vi "Modbus_RTU_Read.vi"(0 "VISA resource name":refnum<visa-resource-name>="COM18", 1 "Serial Config":T1={"baud rate (bps)"=9600, "stop bits"=10, "parity"=0, "flow control"=0, "timeout"=1000, "retries"=1} {"stop bits" items=["1.0"=10, "1.5"=15, "2.0"=20]; "parity" items=["None", "Odd", "Even", "Mark", "Space"]; "flow control" items=["None", "XON/XOFF", "RTS/CTS", "XON/XOFF & RTS/CTS", "DTR/DSR", "XON/XOFF & DTR/DSR"]}, 2 "address":u16=1, 4 "Registers In":u16[](array[numeric])=[1, 0, 2, 0, 0, 0, 0, 0, 0, 9], 5 "error in (no error)":errorcluster, 6 "Function":T2=enum."Read Holding Register03", 7 "Coil Single value":bool=TRUE, 8 "quantity":u16=2, 9 "Register Single Value":u16=100) -> (16 "VALUE":dbl, 19 "error out":errorcluster={"status"=FALSE, "code"=-1073807339, "source"="VISA Read in MB Master.lvlib:MB_ADU_RTU.lvclass:RX ADU.vi:4960001->MB Master.lvlib:MB_Master_Serial.lvclass:Querry.vi:3550001->MB Master.lvlib:Read Holding Registers.vi:2420001->Modbus_RTU_Setting.vi"})   [LabVIEW 2024]
uses:
  Modbus Control.ctl
  <vilib>/Plasmionique/MB Master/MB_Master_Serial/MB_Master_Serial.lvclass
  C:/Program Files (x86)/National Instruments/LabVIEW 2024/vi.lib/Plasmionique/MB Master/MB_Master/MB_Master.lvclass
  <vilib>/Plasmionique/MB Master/MB Master.lvlib
panel:
  out "Registers":u16[](array[numeric])
  out "Coils Outputs":bool[](array[boolean])
  in  "Coils In":bool[](array[boolean])=[TRUE, TRUE, FALSE, FALSE, FALSE, FALSE, FALSE, FALSE, TRUE, TRUE]
  # "Modbus RTU Setting"
  # "Ver1.00"
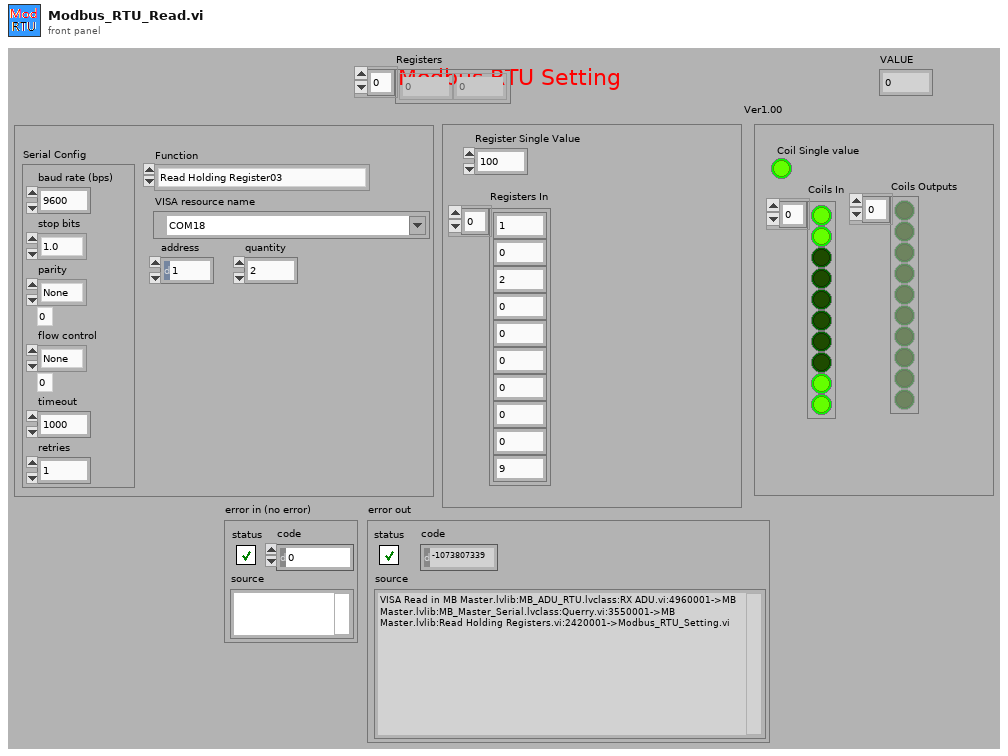
[diagram p1: front panel]
types:
  T1 = cluster{"baud rate (bps)":u32, "stop bits":u16, "parity":u16, "flow control":u16, "timeout":u32, "retries":i32}
  T2 = typedef "Modbus Control.ctl" = enum16{"Read Coils01", "Read Discrete Input02", "Read Holding Register03", "Read Input Registers04", "Write Single Coil05", "Write Single Register06", "Write Multiple Coils15", "Write Multiple Registers16"}
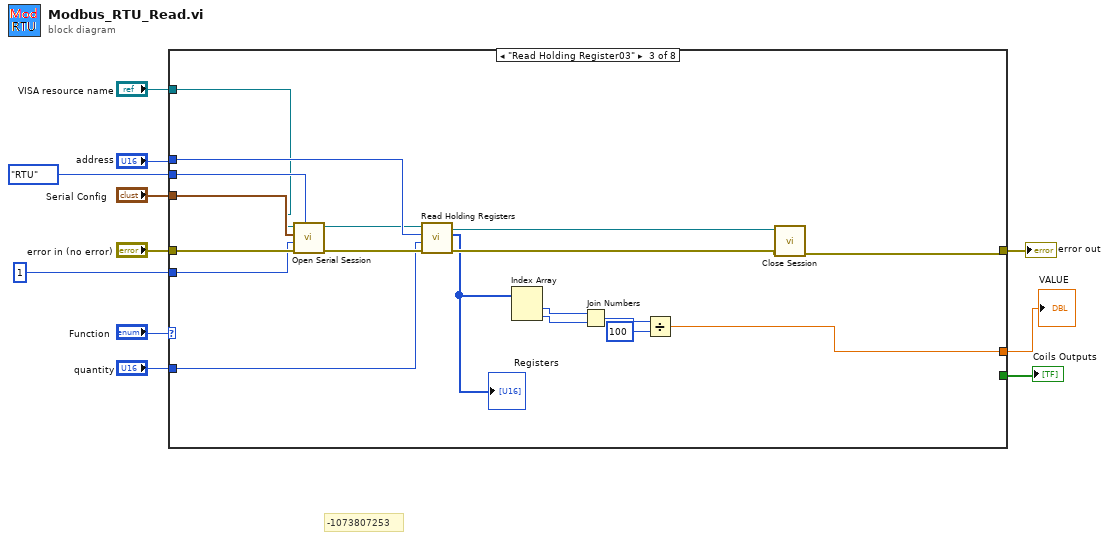
[diagram p0: block diagram]
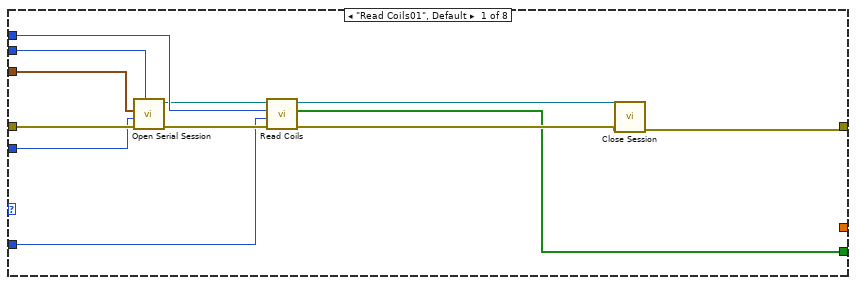
[diagram p2: hidden frame]
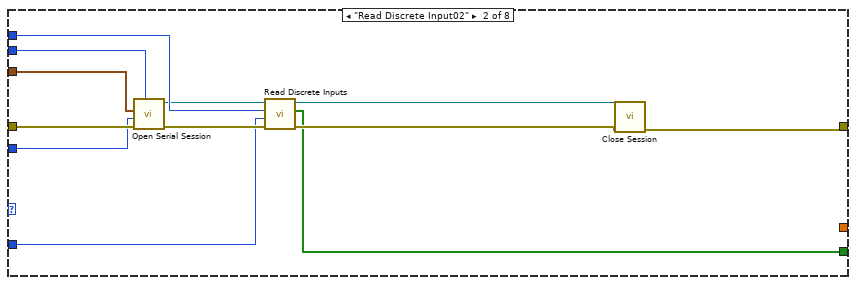
[diagram p3: hidden frame]
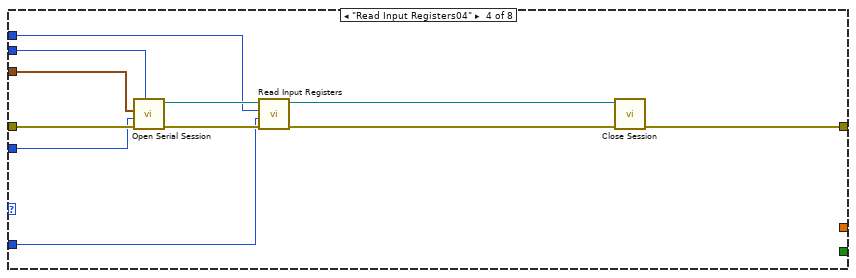
[diagram p4: hidden frame]
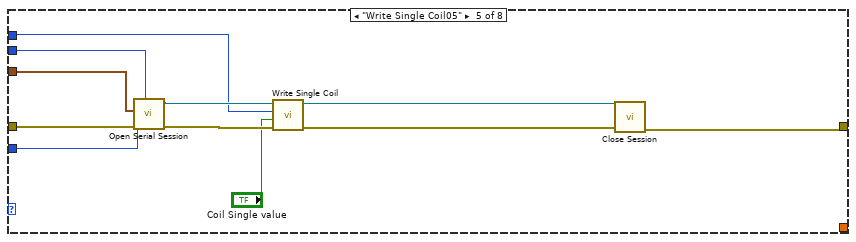
[diagram p5: hidden frame]
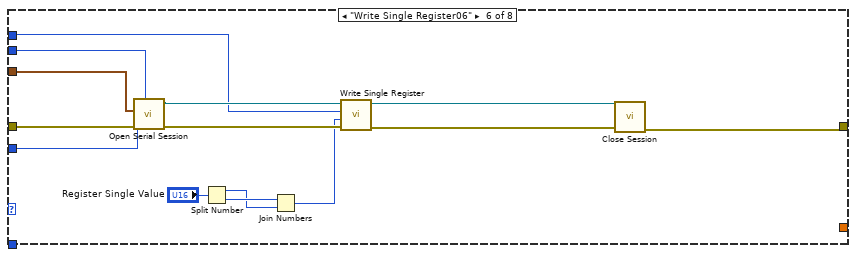
[diagram p6: hidden frame]
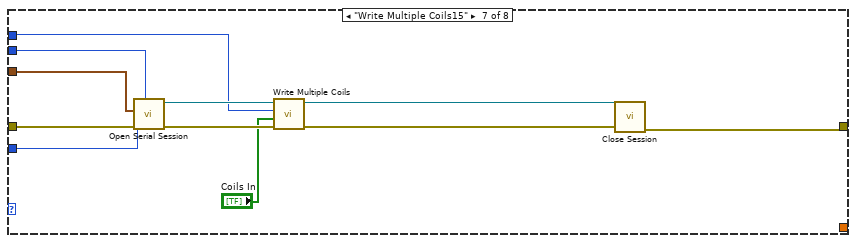
[diagram p7: hidden frame]
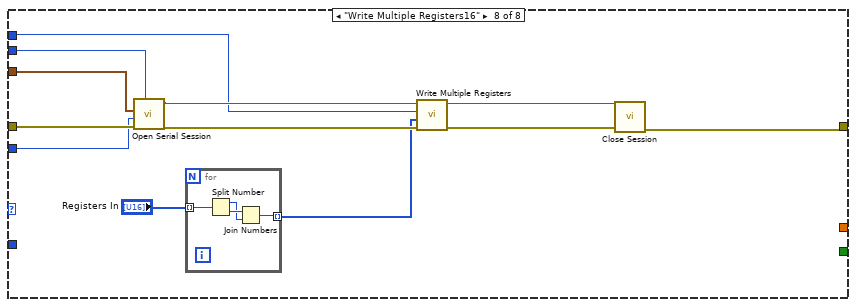
[diagram p8: hidden frame]
diagram:
  # "-1073807253"
  n1 = case shown="\"Read Holding Register03\"" "Function" {
    tunnel: "Serial Config" -> [w22 w34 w51 w63 w74 w88 w99 w111]
    tunnel: "error in (no error)" -> [w23 w35 w52 w64 w75 w89 w100 w112]
    tunnel: [w21 w33 w46 w62 w73 w87 w98 w110] -> w8
    tunnel: "address" -> [w15 w27 w53 w55 w66 w83 w91 w105]
    tunnel: enum16{"RTU", "ASCII"}."RTU" ("Mode (RTU)") -> [w20 w32 w45 w61 w72 w81 w97 w104]
    tunnel: u8 1 ("Slave ID") -> [w19 w31 w44 w60 w71 w80 w96 w103]
    tunnel: "quantity" -> [w16 w28 w43 w54 _ _ _ _]
    tunnel: [w12 w24 _ _ _ _ _ _] -> w3
    tunnel: [_ _ w37 _ _ _ _ _] -> w2
    tunnel: "VISA resource name" -> [_ _ w36 _ _ _ _ _]
    frame "Read Coils01", Default {
      n2 = call <vilib>:"Open Serial Session.vi"("Mode (RTU)"=w20, "Error in"=w23, "Slave ID"=w19, "Serial Config"=w22) -> ("Error out"=w17:errorcluster, "MB_Serial session"=w14:refnum<class "MB_Master_Serial.lvclass">)  [unwired: 6 in]
      n3 = call <vilib>:"Read Coils.vi"("error in (no error)"=w17, "quantity"=w16, "starting address"=w15, "MB session in"=w14) -> ("error out"=w18:errorcluster, "Coils"=w12:bool[], "MB session out"=w13:refnum<class "MB_Master_Serial.lvclass">)  [unwired: 5 in]
      n4 = call-dynamic "Close Session.vi"("error in (no error)"=w18, "MB_Serial session"=w13) -> ("error out"=w21:errorcluster)  [unwired: 9 in]
    }
    frame "Read Discrete Input02" {
      n5 = call <vilib>:"Open Serial Session.vi"("Mode (RTU)"=w32, "Error in"=w35, "Slave ID"=w31, "Serial Config"=w34) -> ("Error out"=w29:errorcluster, "MB_Serial session"=w26:refnum<class "MB_Master_Serial.lvclass">)  [unwired: 6 in]
      n6 = call <vilib>:"Read Discrete Inputs.vi"("error in (no error)"=w29, "quantity"=w28, "starting address"=w27, "MB session in"=w26) -> ("error out"=w30:errorcluster, "Inputs"=w24:bool[], "MB session out"=w25:refnum<class "MB_Master_Serial.lvclass">)  [unwired: 5 in]
      n7 = call-dynamic "Close Session.vi"("error in (no error)"=w30, "MB_Serial session"=w25) -> ("error out"=w33:errorcluster)  [unwired: 9 in]
    }
    frame "Read Holding Register03" {
      n8 = call <vilib>:"Open Serial Session.vi"("Mode (RTU)"=w45, "Error in"=w52, "Slave ID"=w44, "Serial Config"=w51, "VISA Resource"=w36) -> ("Error out"=w50:errorcluster, "MB_Serial session"=w49:refnum<class "MB_Master_Serial.lvclass">)  [unwired: 5 in]
      n9 = call <vilib>:"Read Holding Registers.vi"("error in (no error)"=w50, "quantity"=w43, "starting address"=w53, "MB session in"=w49) -> ("error out"=w48:errorcluster, "Registers"=w42:u16[], "MB session out"=w47:refnum<class "MB_Master_Serial.lvclass">)  [unwired: 5 in]
      "Registers" <- w42
      n10 = Index Array(array=w42) -> (element #1=w41:u16, element #2=w40:u16)  [unwired: 2 in]
      n11 = Join Numbers(hi=w41, lo=w40) -> ((hi.lo)=w39:u32)
      n12 = Divide(x=w39, y=u32 100) -> (x/y=w37:dbl)
      n13 = call-dynamic "Close Session.vi"("error in (no error)"=w48, "MB_Serial session"=w47) -> ("error out"=w46:errorcluster)  [unwired: 9 in]
    }
    frame "Read Input Registers04" {
      n14 = call <vilib>:"Open Serial Session.vi"("Mode (RTU)"=w61, "Error in"=w64, "Slave ID"=w60, "Serial Config"=w63) -> ("Error out"=w58:errorcluster, "MB_Serial session"=w57:refnum<class "MB_Master_Serial.lvclass">)  [unwired: 6 in]
      n15 = call <vilib>:"Read Input Registers.vi"("error in (no error)"=w58, "quantity"=w54, "starting address"=w55, "MB session in"=w57) -> ("error out"=w59:errorcluster, "MB session out"=w56:refnum<class "MB_Master_Serial.lvclass">)  [unwired: 5 in, 1 out]
      n16 = call-dynamic "Close Session.vi"("error in (no error)"=w59, "MB_Serial session"=w56) -> ("error out"=w62:errorcluster)  [unwired: 9 in]
    }
    frame "Write Single Coil05" {
      n17 = call <vilib>:"Open Serial Session.vi"("Mode (RTU)"=w72, "Error in"=w75, "Slave ID"=w71, "Serial Config"=w74) -> ("Error out"=w69:errorcluster, "MB_Serial session"=w68:refnum<class "MB_Master_Serial.lvclass">)  [unwired: 6 in]
      n18 = call <vilib>:"Write Single Coil.vi"("error in (no error)"=w69, "value"="Coil Single value", "address"=w66, "MB session in"=w68) -> ("error out"=w70:errorcluster, "MB session out"=w67:refnum<class "MB_Master_Serial.lvclass">)  [unwired: 6 in]
      n19 = call-dynamic "Close Session.vi"("error in (no error)"=w70, "MB_Serial session"=w67) -> ("error out"=w73:errorcluster)  [unwired: 9 in]
    }
    frame "Write Single Register06" {
      n20 = call <vilib>:"Open Serial Session.vi"("Mode (RTU)"=w81, "Error in"=w89, "Slave ID"=w80, "Serial Config"=w88) -> ("Error out"=w82:errorcluster, "MB_Serial session"=w84:refnum<class "MB_Master_Serial.lvclass">)  [unwired: 6 in]
      n21 = Split Number(x="Register Single Value") -> (hi(x)=w77:u8, lo(x)=w79:u8)
      n22 = Join Numbers(hi=w79, lo=w77) -> ((hi.lo)=w76:u16)
      n23 = call <vilib>:"Write Single Register.vi"("error in (no error)"=w82, "value"=w76, "address"=w83, "MB session in"=w84) -> ("error out"=w86:errorcluster, "MB session out"=w85:refnum<class "MB_Master_Serial.lvclass">)  [unwired: 6 in]
      n24 = call-dynamic "Close Session.vi"("error in (no error)"=w86, "MB_Serial session"=w85) -> ("error out"=w87:errorcluster)  [unwired: 9 in]
    }
    frame "Write Multiple Coils15" {
      n25 = call <vilib>:"Open Serial Session.vi"("Mode (RTU)"=w97, "Error in"=w100, "Slave ID"=w96, "Serial Config"=w99) -> ("Error out"=w94:errorcluster, "MB_Serial session"=w93:refnum<class "MB_Master_Serial.lvclass">)  [unwired: 6 in]
      n26 = call <vilib>:"Write Multiple Coils.vi"("error in (no error)"=w94, "values"="Coils In", "starting address"=w91, "MB session in"=w93) -> ("error out"=w95:errorcluster, "MB session out"=w92:refnum<class "MB_Master_Serial.lvclass">)  [unwired: 6 in]
      n27 = call-dynamic "Close Session.vi"("error in (no error)"=w95, "MB_Serial session"=w92) -> ("error out"=w98:errorcluster)  [unwired: 9 in]
    }
    frame "Write Multiple Registers16" {
      n28 = call <vilib>:"Open Serial Session.vi"("Mode (RTU)"=w104, "Error in"=w112, "Slave ID"=w103, "Serial Config"=w111) -> ("Error out"=w108:errorcluster, "MB_Serial session"=w107:refnum<class "MB_Master_Serial.lvclass">)  [unwired: 6 in]
      n29 = for {
        tunnel: "Registers In" -> [w114] mode=indexing
        tunnel: [w113] -> w101 mode=indexing
        n30 = Split Number(x=w114) -> (hi(x)=w115:u8, lo(x)=w116:u8)
        n31 = Join Numbers(hi=w116, lo=w115) -> ((hi.lo)=w113:u16)
      }
      n32 = call <vilib>:"Write Multiple Registers.vi"("error in (no error)"=w108, "values"=w101, "starting address"=w105, "MB session in"=w107) -> ("error out"=w109:errorcluster, "MB session out"=w106:refnum<class "MB_Master_Serial.lvclass">)  [unwired: 6 in]
      n33 = call-dynamic "Close Session.vi"("error in (no error)"=w109, "MB_Serial session"=w106) -> ("error out"=w110:errorcluster)  [unwired: 9 in]
    }
  }
  "error out" <- w8
  "Coils Outputs" <- w3
  "VALUE" <- w2
